vi "Read P.vi"(8 "error in (no error)":errorcluster, 11 "Update Housekeeping in":refnum<class "Update Housekeeping.lvclass">) -> (0 "error out":errorcluster, 2 "P":dbl[](array[numeric]), 3 "Update Housekeeping out":refnum<class "Update Housekeeping.lvclass">)   [LabVIEW 2014, in "eCRDS Library.lvlib" / "Update Housekeeping.lvclass"]
uses:
  Update Housekeeping.lvclass
  Update Housekeeping.lvclass/Update Housekeeping.ctl
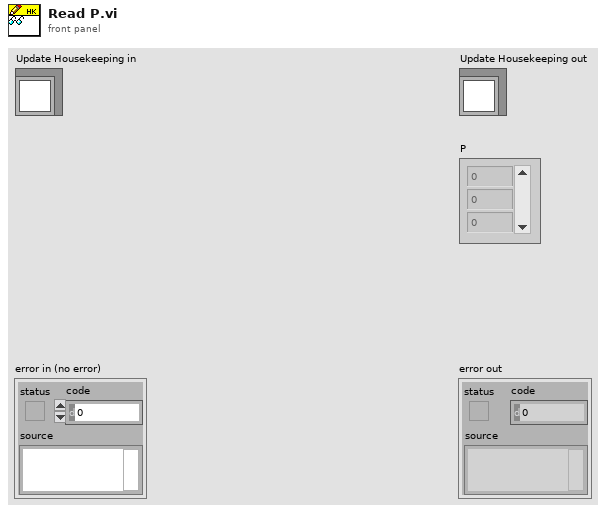
[diagram p1: front panel]
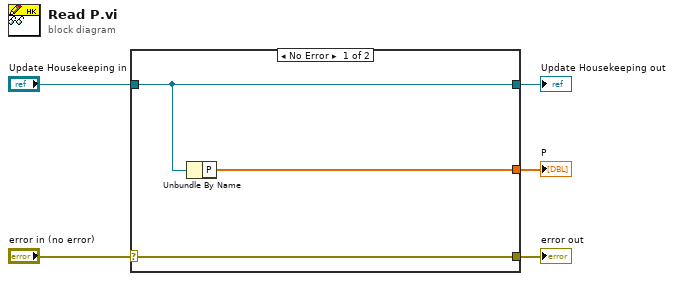
[diagram p0: block diagram]
diagram:
  n1 = case shown="No Error" "error in (no error)" {
    selector: "error in (no error)" -> [w8 w9]
    tunnel: [w8 w9] -> w4
    tunnel: [w7 w10] -> w2
    tunnel: "Update Housekeeping in" -> [w7 w10]
    tunnel: [w6 _] -> w1
    frame No Error {
      n2 = Unbundle By Name(w7) -> ("P"=w6:dbl[])
    }
    frame Error {
    }
  }
  "error out" <- w4
  "Update Housekeeping out" <- w2
  "P" <- w1
